vi "gentec-SOLO-PE.Example.vi"() -> ()   [LabVIEW 2014, in "gentec-SOLO-PE - Driver.lvlib"]
uses:
  gentec-SOLO-PE - Driver.lvlib
  Driver/Type Defs/gentec-SOLO-PE.Configuration Values.ctl
  Driver/Type Defs/gentec-SOLO-PE.Scale.ctl
  Driver/Type Defs/gentec-SOLO-PE.Data Sampling Settings.ctl
  Driver/Type Defs/gentec-SOLO-PE.Statistics Data.ctl
  Driver/Type Defs/gentec-SOLO-PE.Queries with String Answers.ctl
  Driver/Type Defs/gentec-SOLO-PE.Correction Type.ctl
  Driver/Type Defs/gentec-SOLO-PE.Zero Offset.ctl
  Driver/Type Defs/gentec-SOLO-PE.Enable Statistics.ctl
panel:
  out "Configuration after Settings":T1 {"Reference Value" format="%.6f"; "Lower Bond" format="%.6f"; "Upper Bound" format="%.6f"; "Resolution" format="%.7f"; "Max energy (Joulemeter)" format="%.6f"; "Max Power (Joulemeter)" format="%.6f"; "Offset 2" format="%.6f"; "Multiplier 2" format="%.6f"; "Offset 1" format="%.6f"; "Multiplier 1" format="%.6f"; "Zero Offset" format="%.6f"; "Trig Level" format="%.6f"; "Current Scale" items=["Auto", "1 pJ", "3 pJ", "10 pJ", "30 pJ", "100 pJ", "300 pJ", "1 nJ", "3 nJ", "10 nJ", "30 nJ", "100 nJ", "300 nJ", "1 uJ", "3 uJ", "10 uJ", "30 uJ", "100 uJ", "300 uJ", "1 mJ", "3 mJ", "10 mJ", "30 mJ", "100 mJ", "300 mJ", "1 J", "3 J", "10 J", "30 J", "100 J", "300 J", "1 kJ", "3 kJ", "10 kJ", "30 kJ", "100 kJ", "300 kJ", "1 MJ", "3 MJ", "10 MJ", "30 MJ", "100 MJ", "300 MJ"]; "Scale Max Energy" items=["Auto", "1 pJ", "3 pJ", "10 pJ", "30 pJ", "100 pJ", "300 pJ", "1 nJ", "3 nJ", "10 nJ", "30 nJ", "100 nJ", "300 nJ", "1 uJ", "3 uJ", "10 uJ", "30 uJ", "100 uJ", "300 uJ", "1 mJ", "3 mJ", "10 mJ", "30 mJ", "100 mJ", "300 mJ", "1 J", "3 J", "10 J", "30 J", "100 J", "300 J", "1 kJ", "3 kJ", "10 kJ", "30 kJ", "100 kJ", "300 kJ", "1 MJ", "3 MJ", "10 MJ", "30 MJ", "100 MJ", "300 MJ"]; "Scale Min Energy" items=["Auto", "1 pJ", "3 pJ", "10 pJ", "30 pJ", "100 pJ", "300 pJ", "1 nJ", "3 nJ", "10 nJ", "30 nJ", "100 nJ", "300 nJ", "1 uJ", "3 uJ", "10 uJ", "30 uJ", "100 uJ", "300 uJ", "1 mJ", "3 mJ", "10 mJ", "30 mJ", "100 mJ", "300 mJ", "1 J", "3 J", "10 J", "30 J", "100 J", "300 J", "1 kJ", "3 kJ", "10 kJ", "30 kJ", "100 kJ", "300 kJ", "1 MJ", "3 MJ", "10 MJ", "30 MJ", "100 MJ", "300 MJ"]; "Active Sensitivity" format="%.6f"; "Calibration Sensitivity" format="%.6f"}
  out "Corrected Value [J]":dbl
  out "Uncorrected Value [J]":dbl
  out "Statistic Data":T3 {"Uncorrected Value" format="%.6f"; "Rep Rate" format="%.2f"; "Average Power" format="%.6f"; "PTP Stability" format="%.6f"; "RMS Stability" format="%.6f"; "Standard Deviation" format="%.6f"; "Average" format="%.6f"; "Minimum" format="%.6f"; "Maximum" format="%.6f"; "Current Value" format="%.6f"}
  out "All acknoledged?":bool
  out "Data Samling Settings":T4 {"Time Stamp" items=["Off", "On"]; "Total Duration Unit" items=["Period", "Seconds", "Minutes", "Hours", "Days", "Weeks", "Continuous", "# of Points"]; "Total Duration" max=300 step=1; "Sample Period Unit" items=["Seconds", "Minutes", "Hours", "Days", "Weeks", "Pulses"]; "Sample Rate Unit" items=["per Second", "per Minute", "per Hour", "per Day", "% pulses"]; "Sample Rate" max=300 step=1}
  out "Configuration after start":T1 {"Reference Value" format="%.6f"; "Lower Bond" format="%.6f"; "Upper Bound" format="%.6f"; "Resolution" format="%.7f"; "Max energy (Joulemeter)" format="%.6f"; "Max Power (Joulemeter)" format="%.6f"; "Offset 2" format="%.6f"; "Multiplier 2" format="%.6f"; "Offset 1" format="%.6f"; "Multiplier 1" format="%.6f"; "Zero Offset" format="%.6f"; "Trig Level" format="%.6f"; "Current Scale" items=["Auto", "1 pJ", "3 pJ", "10 pJ", "30 pJ", "100 pJ", "300 pJ", "1 nJ", "3 nJ", "10 nJ", "30 nJ", "100 nJ", "300 nJ", "1 uJ", "3 uJ", "10 uJ", "30 uJ", "100 uJ", "300 uJ", "1 mJ", "3 mJ", "10 mJ", "30 mJ", "100 mJ", "300 mJ", "1 J", "3 J", "10 J", "30 J", "100 J", "300 J", "1 kJ", "3 kJ", "10 kJ", "30 kJ", "100 kJ", "300 kJ", "1 MJ", "3 MJ", "10 MJ", "30 MJ", "100 MJ", "300 MJ"]; "Scale Max Energy" items=["Auto", "1 pJ", "3 pJ", "10 pJ", "30 pJ", "100 pJ", "300 pJ", "1 nJ", "3 nJ", "10 nJ", "30 nJ", "100 nJ", "300 nJ", "1 uJ", "3 uJ", "10 uJ", "30 uJ", "100 uJ", "300 uJ", "1 mJ", "3 mJ", "10 mJ", "30 mJ", "100 mJ", "300 mJ", "1 J", "3 J", "10 J", "30 J", "100 J", "300 J", "1 kJ", "3 kJ", "10 kJ", "30 kJ", "100 kJ", "300 kJ", "1 MJ", "3 MJ", "10 MJ", "30 MJ", "100 MJ", "300 MJ"]; "Scale Min Energy" items=["Auto", "1 pJ", "3 pJ", "10 pJ", "30 pJ", "100 pJ", "300 pJ", "1 nJ", "3 nJ", "10 nJ", "30 nJ", "100 nJ", "300 nJ", "1 uJ", "3 uJ", "10 uJ", "30 uJ", "100 uJ", "300 uJ", "1 mJ", "3 mJ", "10 mJ", "30 mJ", "100 mJ", "300 mJ", "1 J", "3 J", "10 J", "30 J", "100 J", "300 J", "1 kJ", "3 kJ", "10 kJ", "30 kJ", "100 kJ", "300 kJ", "1 MJ", "3 MJ", "10 MJ", "30 MJ", "100 MJ", "300 MJ"]; "Active Sensitivity" format="%.6f"; "Calibration Sensitivity" format="%.6f"}
  out "Version":string
  out "Head Name":string
  out "Error":string
  out "No Timeout":bool
  out "No Error!":bool
  out "error out":errorcluster
  in  "VISA Resource Name":refnum<visa-resource-name>="COM4"
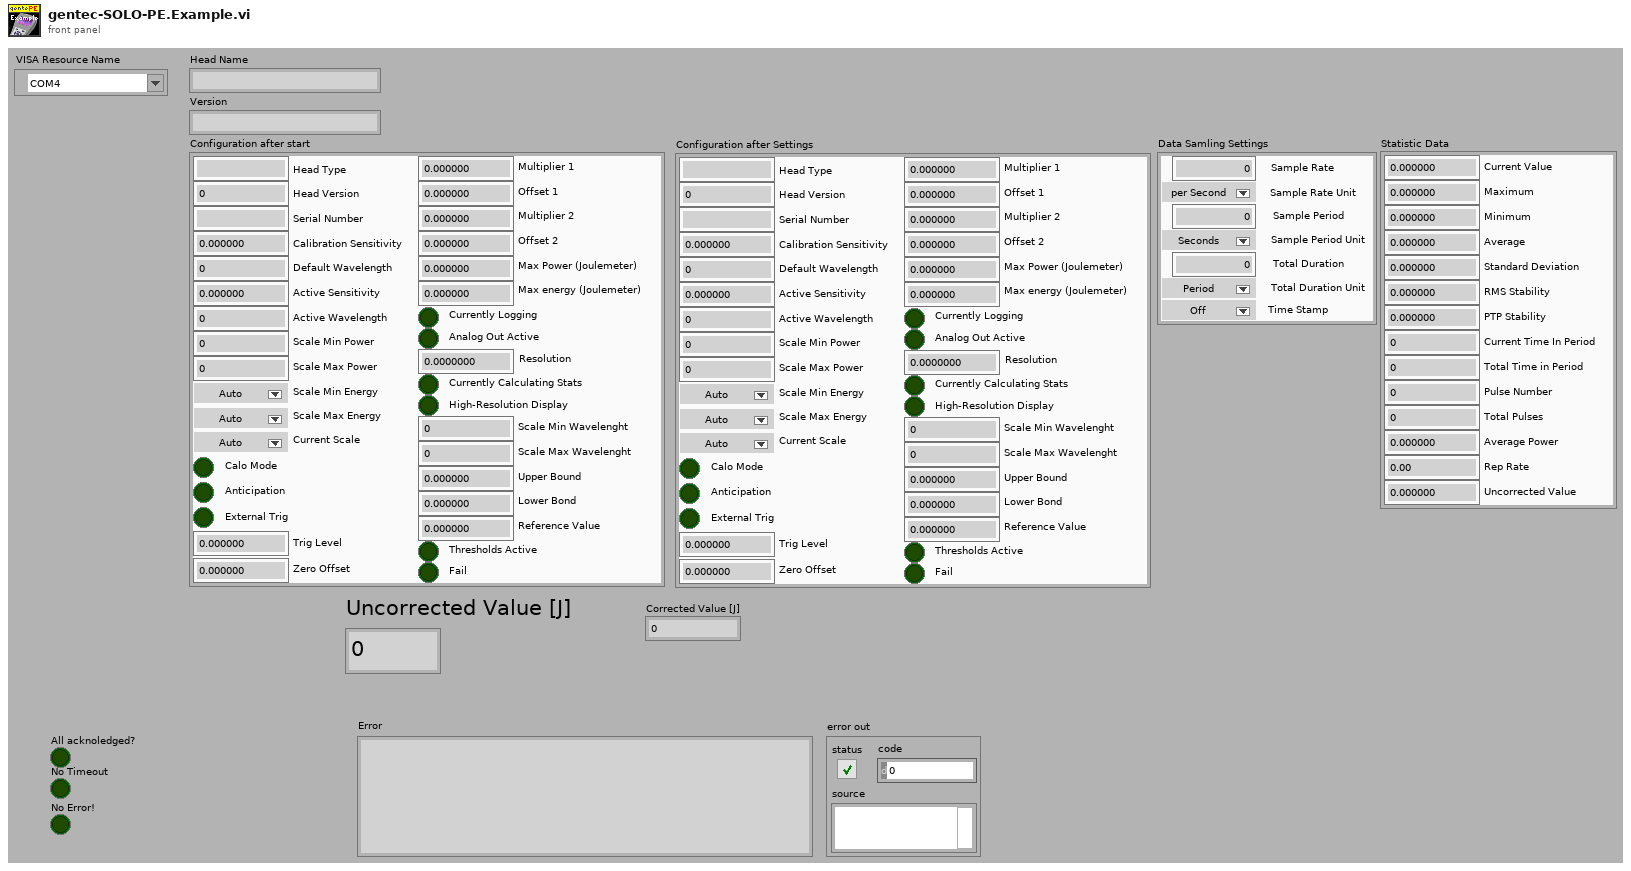
[diagram p1: front panel]
types:
  T1 = typedef "gentec-SOLO-PE - Driver.lvlib/gentec-SOLO-PE.Configuration Values.ctl" = cluster{"Head Type":string, "Head Version":u32, "Serial Number":string, "Calibration Sensitivity":dbl, "Default Wavelength":u32, "Active Sensitivity":dbl, "Active Wavelength":u32, "Scale Min Power":u32, "Scale Max Power":u32, "Scale Min Energy":T2, "Scale Max Energy":T2, "Current Scale":T2, "Calo Mode":bool, "Anticipation":bool, "External Trig":bool, "Trig Level":dbl, "Zero Offset":dbl, "Multiplier 1":dbl, "Offset 1":dbl, "Multiplier 2":dbl, "Offset 2":dbl, "Max Power (Joulemeter)":dbl, "Max energy (Joulemeter)":dbl, "Currently Logging":bool, "Analog Out Active":bool, "Resolution":dbl, "Currently Calculating Stats":bool, "High-Resolution Display":bool, "Scale Min Wavelenght":u32, "Scale Max Wavelenght":u32, "Upper Bound":dbl, "Lower Bond":dbl, "Reference Value":dbl, "Thresholds Active":bool, "Fail":bool}
  T2 = typedef "gentec-SOLO-PE - Driver.lvlib/gentec-SOLO-PE.Scale.ctl" = u32
  T3 = typedef "gentec-SOLO-PE - Driver.lvlib/gentec-SOLO-PE.Statistics Data.ctl" = cluster{"Current Value":dbl, "Maximum":dbl, "Minimum":dbl, "Average":dbl, "Standard Deviation":dbl, "RMS Stability":dbl, "PTP Stability":dbl, "Current Time In Period":u32, "Total Time in Period":u32, "Pulse Number":u32, "Total Pulses":u32, "Average Power":dbl, "Rep Rate":dbl, "Uncorrected Value":dbl}
  T4 = typedef "gentec-SOLO-PE - Driver.lvlib/gentec-SOLO-PE.Data Sampling Settings.ctl" = cluster{"Sample Rate":u32, "Sample Rate Unit":u32, "Sample Period":u32, "Sample Period Unit":u32, "Total Duration":u32, "Total Duration Unit":u32, "Time Stamp":u32}
  T5 = typedef "gentec-SOLO-PE - Driver.lvlib/gentec-SOLO-PE.Enable Statistics.ctl" = u32
  T6 = typedef "gentec-SOLO-PE - Driver.lvlib/gentec-SOLO-PE.Zero Offset.ctl" = u32
  T7 = typedef "gentec-SOLO-PE - Driver.lvlib/gentec-SOLO-PE.Correction Type.ctl" = u16
  T8 = typedef "gentec-SOLO-PE - Driver.lvlib/gentec-SOLO-PE.Queries with String Answers.ctl" = string
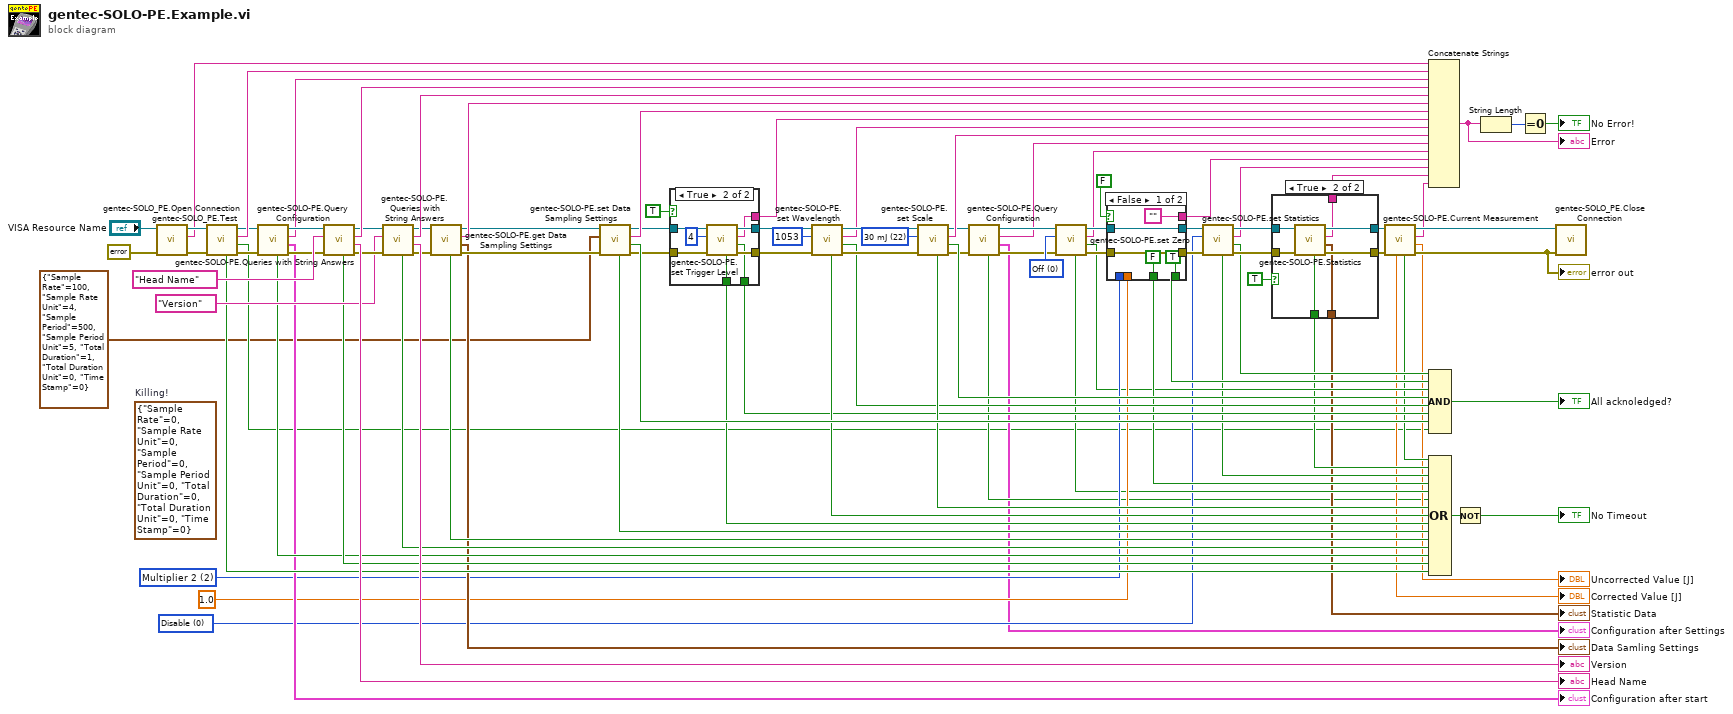
[diagram p0: block diagram]
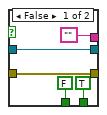
[diagram p2: hidden frame]
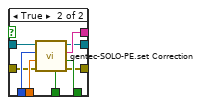
[diagram p3: hidden frame]
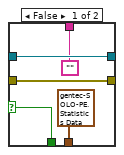
[diagram p4: hidden frame]
diagram:
  (unwired) T4 {"Sample Rate"=0, "Sample Rate Unit"=0, "Sample Period"=0, "Sample Period Unit"=0, "Total Duration"=0, "Total Duration Unit"=0, "Time Stamp"=0}  # Killing!
  w29 = T5 0 items=["Disable", "Enable", "Reset"] ("Enable Statistics")
  w37 = T6 0 items=["Off", "On", "Undo"] ("Zero Offset Operation")
  w44 = T7 2 items=["Multiplier1", "Offset 1", "Multiplier 2", "Offset 2"] ("Correction Type")
  w45 = T2 22 items=["Auto", "1 pJ", "3 pJ", "10 pJ", "30 pJ", "100 pJ", "300 pJ", "1 nJ", "3 nJ", "10 nJ", "30 nJ", "100 nJ", "300 nJ", "1 uJ", "3 uJ", "10 uJ", "30 uJ", "100 uJ", "300 uJ", "1 mJ", "3 mJ", "10 mJ", "30 mJ", "100 mJ", "300 mJ", "1 J", "3 J", "10 J", "30 J", "100 J", "300 J", "1 kJ", "3 kJ", "10 kJ", "30 kJ", "100 kJ", "300 kJ", "1 MJ", "3 MJ", "10 MJ", "30 MJ", "100 MJ", "300 MJ"] ("Scale")
  n1 = call "gentec-SOLO_PE.Open Connection.vi"("error in"=errorcluster {"status"=FALSE, "code"=0, "source"=""} ("error in (no error)"), "VISA resource name in"="VISA Resource Name") -> ("error out"=w97:errorcluster, "Error"=w93:string, "VISA resource name out"=w96:refnum<visa-resource-name>)  [unwired: 3 in]
  n2 = call "gentec-SOLO_PE.Test.vi"("error in (no error)"=w97, "VISA Refnum in"=w96) -> ("error out"=w78:errorcluster, "Acknoledged?"=w2:bool, "Error"=w92:string, "VISA Refnum out"=w76:refnum<visa-resource-name>, "Timeout"=w82:bool)  [unwired: 5 in]
  n3 = call "gentec-SOLO-PE.Query Configuration.vi"("error in (no error)"=w78, "VISA Refnum in"=w76) -> ("error out"=w77:errorcluster, "Configuration"=→"Configuration after start":T1, "Error"=w74:string, "VISA Refnum out"=w75:refnum<visa-resource-name>, "Timeout"=w73:bool)  [unwired: 5 in]
  n4 = call "gentec-SOLO-PE.Queries with String Answers.vi"("error in (no error)"=w77, "Queries with String Answers"=T8 "Head Name", "VISA Refnum in"=w75) -> ("error out"=w87:errorcluster, "Answer"=→"Head Name":string, "Error"=w88:string, "VISA Refnum out"=w86:refnum<visa-resource-name>, "Timeout"=w81:bool)  [unwired: 4 in]
  n5 = call "gentec-SOLO-PE.Queries with String Answers.vi"("error in (no error)"=w87, "Queries with String Answers"=T8 "Version", "VISA Refnum in"=w86) -> ("error out"=w70:errorcluster, "Answer"=→"Version":string, "Error"=w84:string, "VISA Refnum out"=w71:refnum<visa-resource-name>, "Timeout"=w80:bool)  [unwired: 4 in]
  n6 = call "gentec-SOLO-PE.get Data Sampling Settings.vi"("error in (no error)"=w70, "VISA Refnum in"=w71) -> ("error out"=w66:errorcluster, "Data Samling Settings"=→"Data Samling Settings":T4, "Error"=w69:string, "VISA Refnum out"=w67:refnum<visa-resource-name>, "Timeout"=w68:bool)  [unwired: 5 in]
  n7 = call "gentec-SOLO-PE.set Data Sampling Settings.vi"("error in (no error)"=w66, "Data Samling Settings"=T4 {"Sample Rate"=100, "Sample Rate Unit"=4, "Sample Period"=500, "Sample Period Unit"=5, "Total Duration"=1, "Total Duration Unit"=0, "Time Stamp"=0} ("Data Sampling Settings"), "VISA Refnum in"=w67) -> ("error out"=w5:errorcluster, "Acknoledged?"=w64:bool, "Error"=w61:string, "VISA Refnum out"=w4:refnum<visa-resource-name>, "Timeout"=w65:bool)  [unwired: 4 in]
  n8 = case shown="True" TRUE {
    tunnel: [w103 w112] -> w59
    tunnel: [w102 w111] -> w57
    tunnel: ["" w110] -> w55
    tunnel: [FALSE ("Timeout") w109] -> w52
    tunnel: [TRUE ("Acknoledged?") w108] -> w49
    tunnel: w5 -> [w102 w107]
    tunnel: w4 -> [w103 w106]
    frame False {
    }
    frame True {
      n9 = call "gentec-SOLO-PE.set Trigger Level.vi"("error in (no error)"=w107, "Trigger Level (2%)"=u32 4, "VISA Refnum in"=w106) -> ("error out"=w111:errorcluster, "Acknoledged?"=w108:bool, "Error"=w110:string, "VISA Refnum out"=w112:refnum<visa-resource-name>, "Timeout"=w109:bool)  [unwired: 4 in]
    }
  }
  n10 = call "gentec-SOLO-PE.set Wavelength.vi"("error in (no error)"=w57, "Wavelength [nm]"=u32 1053, "VISA Refnum in"=w59) -> ("error out"=w56:errorcluster, "Acknoledged?"=w48:bool, "Error"=w54:string, "VISA Refnum out"=w58:refnum<visa-resource-name>, "Timeout"=w51:bool)  [unwired: 4 in]
  n11 = call "gentec-SOLO-PE.set Scale.vi"("error in (no error)"=w56, "Scale"=w45, "VISA Refnum in"=w58) -> ("error out"=w13:errorcluster, "Acknoledged?"=w47:bool, "Error"=w53:string, "VISA Refnum out"=w11:refnum<visa-resource-name>, "Timeout"=w50:bool)  [unwired: 4 in]
  n12 = call "gentec-SOLO-PE.Query Configuration.vi"("error in (no error)"=w13, "VISA Refnum in"=w11) -> ("error out"=w12:errorcluster, "Configuration"=→"Configuration after Settings":T1, "Error"=w9:string, "VISA Refnum out"=w10:refnum<visa-resource-name>, "Timeout"=w8:bool)  [unwired: 5 in]
  n13 = call "gentec-SOLO-PE.set Zero.vi"("error in (no error)"=w12, "Zero Offset Operation"=w37, "VISA Refnum in"=w10) -> ("error out"=w38:errorcluster, "Acknoledged?"=w35:bool, "Error"=w34:string, "VISA Refnum out"=w39:refnum<visa-resource-name>, "Timeout"=w36:bool)  [unwired: 4 in]
  n14 = case shown="False" FALSE {
    tunnel: w44 -> [_ w126]
    tunnel: 1.0 ("Correction Value") -> [_ w125]
    tunnel: ["" w124] -> w42
    tunnel: [TRUE ("Acknoledged?") w123] -> w41
    tunnel: [FALSE ("Timeout") w122] -> w40
    tunnel: w39 -> [w117 w121]
    tunnel: w38 -> [w116 w120]
    tunnel: [w117 w119] -> w33
    tunnel: [w116 w118] -> w31
    frame False {
    }
    frame True {
      n15 = call "gentec-SOLO-PE.set Correction.vi"("error in (no error)"=w120, "Correction Value"=w125, "Correction Type"=w126, "VISA Refnum in"=w121) -> ("error out"=w118:errorcluster, "Acknoledged?"=w123:bool, "Error"=w124:string, "VISA Refnum out"=w119:refnum<visa-resource-name>, "Timeout"=w122:bool)  [unwired: 3 in]
    }
  }
  n16 = call "gentec-SOLO-PE.set Statistics.vi"("error in (no error)"=w31, "Enable Statistics"=w29, "VISA Refnum in"=w33) -> ("error out"=w32:errorcluster, "Acknoledged?"=w27:bool, "Error"=w28:string, "VISA Refnum out"=w30:refnum<visa-resource-name>, "Timeout"=w26:bool)  [unwired: 4 in]
  n17 = case shown="True" TRUE {
    selector: TRUE -> [w128 _]
    tunnel: w32 -> [w131 w138]
    tunnel: [w131 w137] -> w18
    tunnel: w30 -> [w130 w136]
    tunnel: [w130 w135] -> w20
    tunnel: ["" w134] -> w25
    tunnel: [w128 w133] -> w24
    tunnel: [T3 {"Current Value"=0.0, "Maximum"=0.0, "Minimum"=0.0, "Average"=0.0, "Standard Deviation"=0.0, "RMS Stability"=0.0, "PTP Stability"=0.0, "Current Time In Period"=0, "Total Time in Period"=0, "Pulse Number"=0, "Total Pulses"=0, "Average Power"=0.0, "Rep Rate"=0.0, "Uncorrected Value"=0.0} ("Statistic Data") w132] -> w23
    frame False {
    }
    frame True {
      n18 = call "gentec-SOLO-PE.Statistics.vi"("error in (no error)"=w138, "VISA Refnum in"=w136) -> ("error out"=w137:errorcluster, "Statistic Data"=w132:T3, "Error"=w134:string, "VISA Refnum out"=w135:refnum<visa-resource-name>, "Timeout"=w133:bool)  [unwired: 5 in]
    }
  }
  "Statistic Data" <- w23
  n19 = call "gentec-SOLO-PE.Current Measurement.vi"("error in (no error)"=w18, "VISA Refnum in"=w20) -> ("error out"=w19:errorcluster, "Uncorrected Value [J]"=→"Uncorrected Value [J]":dbl, "Error"=w17:string, "VISA Refnum out"=w21:refnum<visa-resource-name>, "Timeout"=w16:bool, "Corrected Value [J]"=→"Corrected Value [J]":dbl)  [unwired: 4 in]
  "error out" <- w19
  n20 = Concatenate Strings(w93, w92, w74, w88, w84, w69, w61, w55, w54, w53, w9, w34, w42, w28, w25, w17) -> (w91:string)
  "Error" <- w91
  n21 = Compound Arithmetic op=AND(w27, w41, w35, w47, w48, w49, w64, w2) -> (→"All acknoledged?":bool)
  n22 = Compound Arithmetic op=OR(w16, w24, w26, w40, w36, w8, w50, w51, w52, w65, w68, w80, w73, w81, w82) -> (w79:bool)
  n23 = Not(x=w79) -> (.not. x?=→"No Timeout":bool)
  n24 = String Length(string=w91) -> (length=w95:i32)
  n25 = Equal To 0?(x=w95) -> (x = 0?=→"No Error!":bool)
  n26 = call "gentec-SOLO_PE.Close Connection.vi"("error in"=w19, "VISA resource name in"=w21) -> ()  [unwired: 5 in, 1 out]
